vi "PH_OceanOpticsSpectrometer.Set Trigger.vi"(0 "i ref in":refnum<vi>, 5 "error in (no error)":errorcluster) -> (14 "i ref out":refnum<vi>, 19 "error out":errorcluster)   [LabVIEW 2014, in "PH_OceanOpticsSpectrometer.lvlib"]
doc: "This VI sets the trigger configuration."
uses:
  PH_OceanOpticsSpectrometer.lvlib
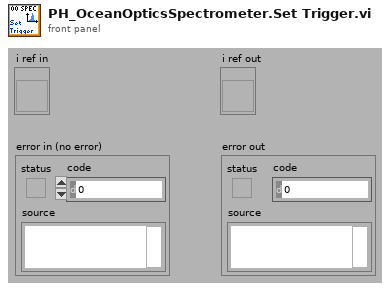
[diagram p1: front panel]
types:
  T1 = typedef "PH_OceanOpticsSpectrometer.lvlib/PH_OceanOpticsSpectrometer.i attribute.ctl" = cluster{"GUI Refs":cluster{"Delete":refnum<vi>, "Spectrum":refnum<vi>, "Display Width":refnum<vi>, "Display Center":refnum<vi>, "Save":refnum<vi>, "Integration time":refnum<vi>, "center wavelength":refnum<vi>, "width":refnum<vi>, "Wanted Trigger Mode":refnum<vi>, "Current Trigger Mode":refnum<vi>, "Trigger Info":refnum<vi>, "Model":refnum<vi>, "Driver":refnum<vi>, "Firmware":refnum<vi>}, "Display":cluster{"Width":dbl, "Center":dbl}, "VISA resource name":refnum<visa-resource-name>, "Integration time [ms]":cluster{"Current Value":u16, "Wanted Value":u16}, "Trigger":cluster{"Current value":T2, "Wanted value":T2}, "Default VISA Timeout":u32, "Last Data":cluster{"Wavelength Bins":dbl[], "Spectrum by Pixels":dbl[]}}
  T2 = typedef "PH_OceanOpticsSpectrometer.lvlib/PH_OceanOpticsSpectrometer.Trigger.ctl" = enum32{"External", "Normal"}
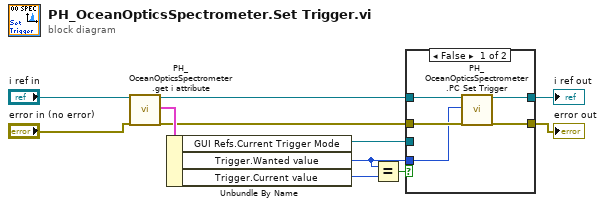
[diagram p0: block diagram]
diagram:
  n1 = call "PH_OceanOpticsSpectrometer.get i attribute.vi"("i ref in"="i ref in", "error in (no error)"="error in (no error)") -> ("i ref out"=w2:refnum<vi>, "i attribute"=w11:T1, "error out"=w1:errorcluster)  [unwired: 15 in]
  n2 = Unbundle By Name(w11) -> ("GUI Refs.Current Trigger Mode"=w3:refnum<vi>, "Trigger.Wanted value"=w4:T2, "Trigger.Current value"=w6:T2)
  n3 = Equal?(x=w4, y=w6) -> (x = y?=w5:bool)
  n4 = case shown="False" w5 {
    tunnel: [w16 w18] -> w10
    tunnel: [w15 w17] -> w8
    tunnel: w2 -> [w14 w17]
    tunnel: w1 -> [w13 w18]
    tunnel: w4 -> [w12 _]
    tunnel: w3 -> [_ _]
    frame False {
      n5 = call "PH_OceanOpticsSpectrometer.PC Set Trigger.vi"("VI in"=w14, "Wanted Trigger"=w12, "error in (no error)"=w13) -> ("VI out"=w15:refnum<vi>, "error out"=w16:errorcluster)  [unwired: 15 in]
    }
    frame True {
    }
  }
  "error out" <- w10
  "i ref out" <- w8
